vi "RelayQueueName.vi"(8 "error in (no error)":errorcluster, 10 "id":string) -> (0 "error out":errorcluster, 3 "queueName":string)   [LabVIEW 2026, in "Lumberjack.lvlib" / "RelayAppender.lvclass"]
doc: "Derives the relay queue's name from the appender id, so Init (the creator) and OpenSink (the reconnector) always obtain the same named queue. Prefixes the id with a fixed namespace so the queue can't collide with unrelated named queues in the host process. Pure, no state."
uses:
  RelayAppender.lvclass
  RelayAppender.lvclass/RelayAppender.ctl
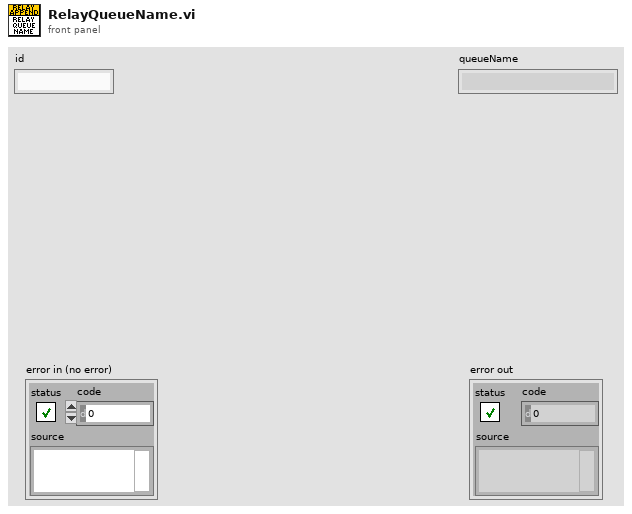
[diagram p1: front panel]
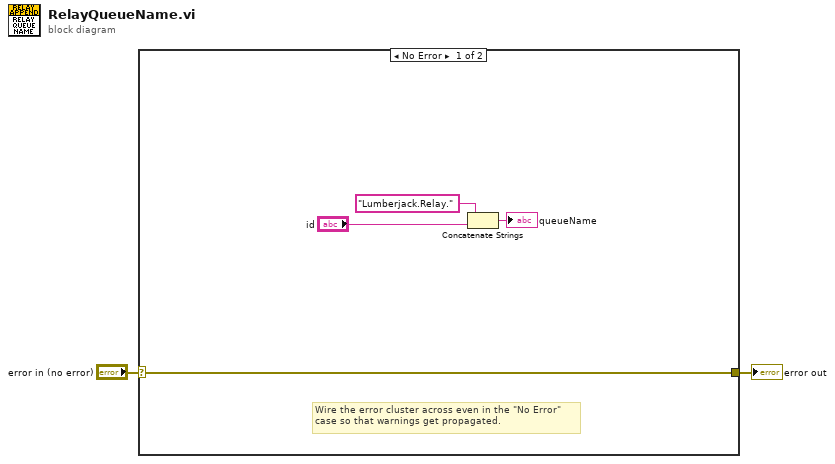
[diagram p0: block diagram]
diagram:
  n1 = case shown="No Error" "error in (no error)" {
    selector: "error in (no error)" -> [w3 w7]
    tunnel: [w3 w7] -> w1
    frame No Error {
      # "Wire the error cluster across even in the \"No Error\"\ncase so that warnings get propagated."
      n2 = Concatenate Strings("Lumberjack.Relay." ("string"), "id") -> (→"queueName":string)
    }
    frame Error {
    }
  }
  "error out" <- w1
